vi "Handle Last Ack.vi"(8 "error in (no error)":errorcluster, 10 "Last Ack":refnum<class "Last Ack.lvclass">, 11 "Actor in":refnum<class "Actor.lvclass">) -> (0 "error out":errorcluster, 3 "Actor out":refnum<class "Actor.lvclass">)   [LabVIEW 2020, in "Actor Framework.lvlib" / "Actor.lvclass"]
doc: "(<B>Filename</B>: Actor Framework.lvlib:Actor.lvclass:Handle Last Ack.vi)\n\nThis VI is a wrapper around Handle Last Ack Core.vi. This wrapper is invoked by the Do method of the Last Ack class."
uses:
  Actor.lvclass
  LastAck/Last Ack.lvclass
  Actor.lvclass/Actor.ctl
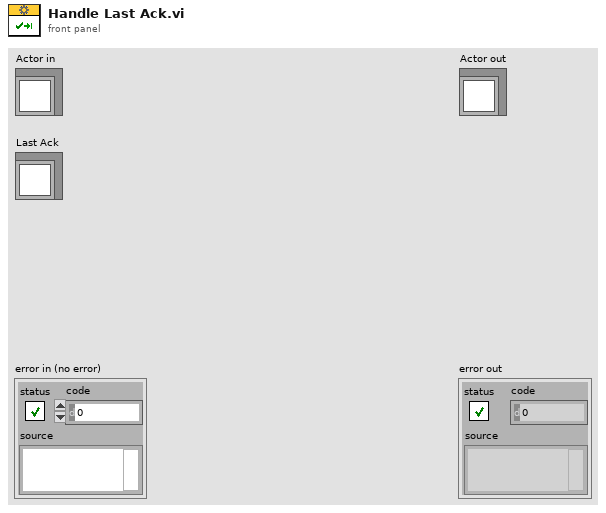
[diagram p1: front panel]
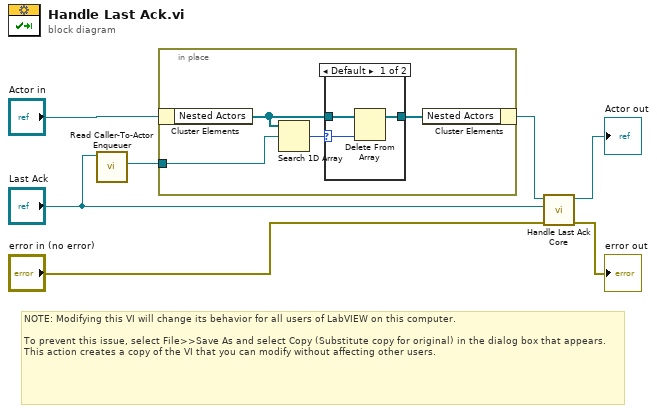
[diagram p0: block diagram]
diagram:
  # "NOTE: Modifying this VI will change its behavior for all users of LabVIEW on this computer.\n\nTo prevent this issue, select File>>Save As and select Copy (Substitute copy for original) in the dialog box that appears. This action creates a copy of the VI that you can modify without affecting other users."
  n1 = call "Read Caller-To-Actor Enqueuer.vi"("Last Ack"="Last Ack") -> ("Caller-to-Actor Enqueuer"=w2:refnum<class "Message Enqueuer.lvclass">)  [unwired: 10 in]
  n2 = in-place {
    in-place-border: w2 -> [w11]
    n3 = in-place-cluster #1("Actor in") -> ("Nested Actors"=w8:refnum<class "Message Enqueuer.lvclass">[])
    n4 = Search 1D Array(1D array=w8, element=w11) -> (index of element=w10:i32)  [unwired: 1 in]
    n5 = case shown="Default" w10 {
      selector: w10 -> [w12 _]
      tunnel: [w13 w15] -> w9
      tunnel: w8 -> [w14 w15]
      frame Default {
        n6 = Delete From Array(array=w14, index=w12) -> (array with subset deleted=w13:refnum<class "Message Enqueuer.lvclass">[])  [unwired: 1 in, 1 out]
      }
      frame -1 {
      }
    }
    n7 = in-place-cluster #1("Nested Actors"=w9) -> (w1:refnum<class "Actor.lvclass">)
  }
  n8 = call-dynamic "Handle Last Ack Core.vi"("error in (no error)"="error in (no error)", "Last Ack"="Last Ack", "Actor in"=w1) -> ("error out"=→"error out":errorcluster, "Actor out"=→"Actor out":refnum<class "Actor.lvclass">)  [unwired: 3 in]
